vi "Example Test 2.vi"() -> ()   [LabVIEW 2014]
uses:
  MPU6050LibVector.ctl
  Arduino MPU6050.lvlib
panel:
  out "Vector 5":T1
  out "Vector 4":T1
  out "temp":dbl
  out "Vector 3":T1
  out "Vector 2":T1
  out "Vector":T1
  in  "error in":errorcluster
  out "error out":errorcluster
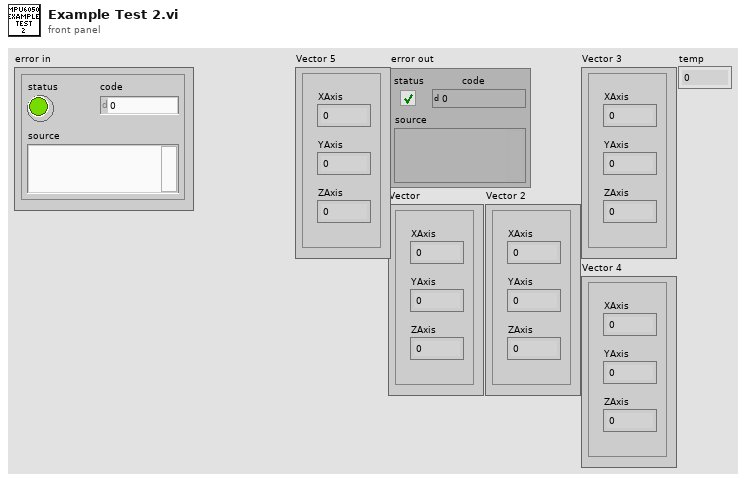
[diagram p1: front panel]
types:
  T1 = typedef "Arduino MPU6050.lvlib/MPU6050LibVector.ctl" = cluster{"XAxis":dbl, "YAxis":dbl, "ZAxis":dbl}
  T2 = enum16{"MPU6050_RANGE_2G", "MPU6050_RANGE_4G", "MPU6050_RANGE_8G", "MPU6050_RANGE_16G"}
  T3 = enum16{"MPU6050_SCALE_250DPS", "MPU6050_SCALE_500DPS", "MPU6050_SCALE_1000DPS", "MPU6050_SCALE_2000DPS"}
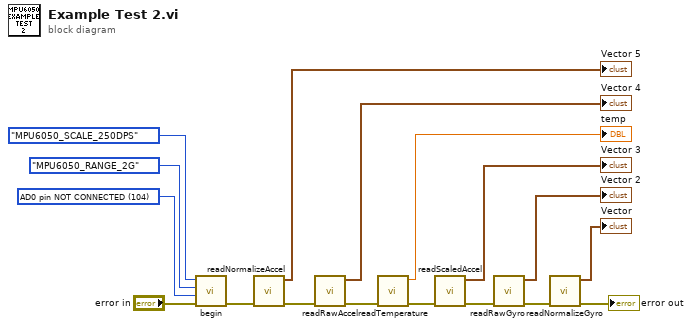
[diagram p0: block diagram]
diagram:
  w1 = u16 104 items=["AD0 pin NOT CONNECTED"=104, "AD0 connect to Vcc"=105] ("address")
  n1 = call "begin.vi"("Error In"="error in", "address"=w1, "range"=T2."MPU6050_RANGE_2G", "scale"=T3."MPU6050_SCALE_250DPS") -> ("Error Out"=w16:errorcluster)  [unwired: 7 in]
  n2 = call "readNormalizeAccel.vi"("error in (no error)"=w16) -> ("error out"=w15:errorcluster, "Vector"=→"Vector 5":T1)  [unwired: 9 in]
  n3 = call "readRawAccel.vi"("error in (no error)"=w15) -> ("error out"=w14:errorcluster, "Vector"=→"Vector 4":T1)  [unwired: 9 in]
  n4 = call "readTemperature.vi"("error in (no error)"=w14) -> ("error out"=w13:errorcluster, "temp"=→"temp":dbl)  [unwired: 9 in]
  n5 = call "readScaledAccel.vi"("error in (no error)"=w13) -> ("error out"=w12:errorcluster, "Vector"=→"Vector 3":T1)  [unwired: 9 in]
  n6 = call "readRawGyro.vi"("error in (no error)"=w12) -> ("error out"=w11:errorcluster, "Vector"=→"Vector 2":T1)  [unwired: 9 in]
  n7 = call "readNormalizeGyro.vi"("error in (no error)"=w11) -> ("error out"=→"error out":errorcluster, "Vector"=→"Vector":T1)  [unwired: 9 in]
